vi "TurnOff.vi"(8 "error in (no error)":errorcluster, 11 "PSU in":refnum<class "PSU.lvclass">) -> (0 "error out":errorcluster, 3 "PSU out":refnum<class "PSU.lvclass">)   [LabVIEW 2014, in "PSU.lvclass"]
uses:
  PSU.lvclass
  PSU.lvclass/PSU.ctl
  Write On.vi
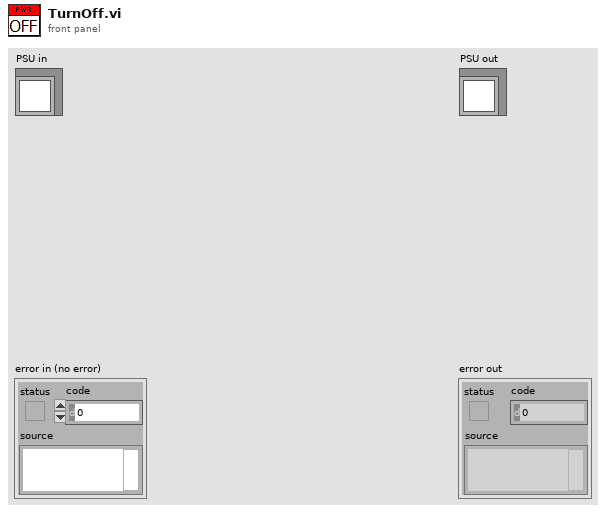
[diagram p1: front panel]
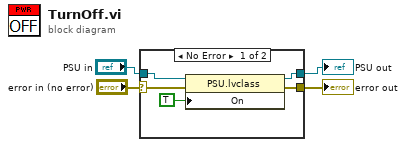
[diagram p0: block diagram]
diagram:
  n1 = case shown="No Error" "error in (no error)" {
    selector: "error in (no error)" -> [w7 w10]
    tunnel: "PSU in" -> [w5 w11]
    tunnel: [w9 w11] -> w2
    tunnel: [w8 w10] -> w1
    frame No Error {
      n2 = property class="PSU.lvclass"(reference=w5, error in=w7, "On"=TRUE) -> (reference out=w9:refnum<class "PSU.lvclass">, error out=w8:errorcluster)
    }
    frame Error {
    }
  }
  "error out" <- w1
  "PSU out" <- w2
